vi "TrapControllers.vi"() -> ()   [LabVIEW 2016]
doc: "I. Description:\nThis example demonstrates how to continuously output a waveform using an internal sample clock. The automatic regeneration of data has been disabled, so new data has to be provided throughout the duration of the continuous Analog Output operation. This allows the generation of any arbitrary frequency as this VI computes new data for each iteration of the loop, maintaining phase continuity of the signal. The regeneration of data has also been adjusted so that the newest data is output as quickly as possible; thus reducing the lag between the changing of the data and the output of that data.\n\nII. Instructions for Running:\n1. Select the Physical Channel to correspond to where your signal is output on the DAQ device.\n2. Enter the Minimum and Maximum Voltage range.\n3. Specify the desired Sample Clock Rate of the output Waveform. Higher sample clock rates will produce a smoother waveform.\n4. Manually specify the Analog Output buffer size, in number of samples. A larger buffer would help non-regenerative operations avoid errors due to occasional high CPU load. \nNote: \nThe Analog Output buffer has to be at least as big as the amount of data being written to the board per iteration. The recommended buffer size would be at least twice the amount of data being written to the board per iteration.\n5. Enter the Waveform Information. See the documentation of the Basic Function Generator SubVI for information on each parameter.\n\nIII. Block Diagram Steps:\n1. Create an Analog Output Voltage channel.\n2. Configure the task to prohibit the automatic regeneration of data.\n2a. Set the transfer condition to Less than Full. Allows for more rapid updates of Output Buffer.\n3. Call the DAQmx (Sample Clock) VI to set the sample clock rate. Additionally, set the sample mode to Continuous.\n4. Read the actual sample clock rate (eventually coerced depending on the hardware used). \n5. Compute the desired waveform, using the buffer size and the actual update rate. This VI keeps track of the phase of the waveform to ensure that the generated signal is continuous.\n6. Write the waveform to the output buffer. \n7a. Call the Start VI. This is only needed when the loop is executed for the first time.\n7b. Do nothing.\n8. Loop continuously until user presses the Stop button. Every iteration computes and writes a new waveform to the buffer.\n9. Call the Clear Task VI to clear the Task.\n10. Use the popup dialog box to display an error or warning if any.\n\nIV. I/O Connections Overview:\nMake sure your signal output terminal matches the Physical Channel I/O Control. For further connection information, refer to your hardware reference manual."
uses:
  TrapControllers/PI_PZT controller/PZT_oscillation_stop.vi
panel:
  out "PZT_manual_on":bool
  in  "PZT_oscillation_stop":bool
  out "Loop stop":bool
  out "Numeric":i32
  in  "PZT_Amplitude":dbl=10.0 caption="Amp (nm)" min=0.0 max=100.0 step=1.0 format="%.2f"
  in  "PZT_Frequency":dbl=1.0 caption="Freq (Hz)" min=0.0 max=100.0 step=1.0 format="%.2f"
  in  "PZT_Waveform":T1(ring) caption="Waveform"
  in  "PZT_Axis":enum16{"X-axis", "Y-axis", "Z-axis"}(ring) caption="Axis"
  in  "PZT_oscillation_start":bool caption="Start"
  in  "PZTZ_move":i32=15000 caption="Z"
  in  "PZTY_move":i32=25000 caption="Y"
  in  "PZTX_move":i32=25000 caption="X"
  out "PZTZ_Vin":dbl format="%.4f"
  out "PZTY_Vin":dbl format="%.4f"
  out "PZTX_Vin":dbl format="%.4f"
  out "PZT_Z":i32 caption="Z"
  out "PZT_Y":i32 caption="Y"
  out "PZT_X":i32 caption="X"
  in  "PZT_Move":bool
  out "PZT_Caution":bool caption="Caution"
  in  "PZT_Time":u32=100 caption="Time \n(ms)" max=1000 step=1
  in  "PZT_Step":i32=10 caption="Step \n(nm)" min=0 max=1000 step=1
  in  "PZT_Center":bool
  in  "PZT_Z-":bool
  in  "PZT_Z+":bool
  in  "PZT_Y-":bool
  in  "PZT_Y+":bool
  in  "PZT_X+":bool
  in  "PZT_X-":bool
  out "PZT_ON":bool
  in  "PZT_Start":bool
  out "PZT_Num":i32
  in  "PZT_Stop":bool
  in  "stop 5":bool
  out "Numeric 5":i32
  in  "OK Button 6":bool
  out "OK Button 5":bool
  out "OK Button 4":bool
  in  "stop 2":bool
  out "Numeric 4":i32
  in  "OK Button 2":bool
  in  "STOP":bool
  # "Stop sub-programs first >> STOP PROGRAM"
  # "Servo should be ON."
  # "Manual"
  # "Oscillation"
  # "LED"
  # "Trap Laser"
  # "Move to"
  # "Pos (nm)"
  # "Vin (V)"
  # "PZT"
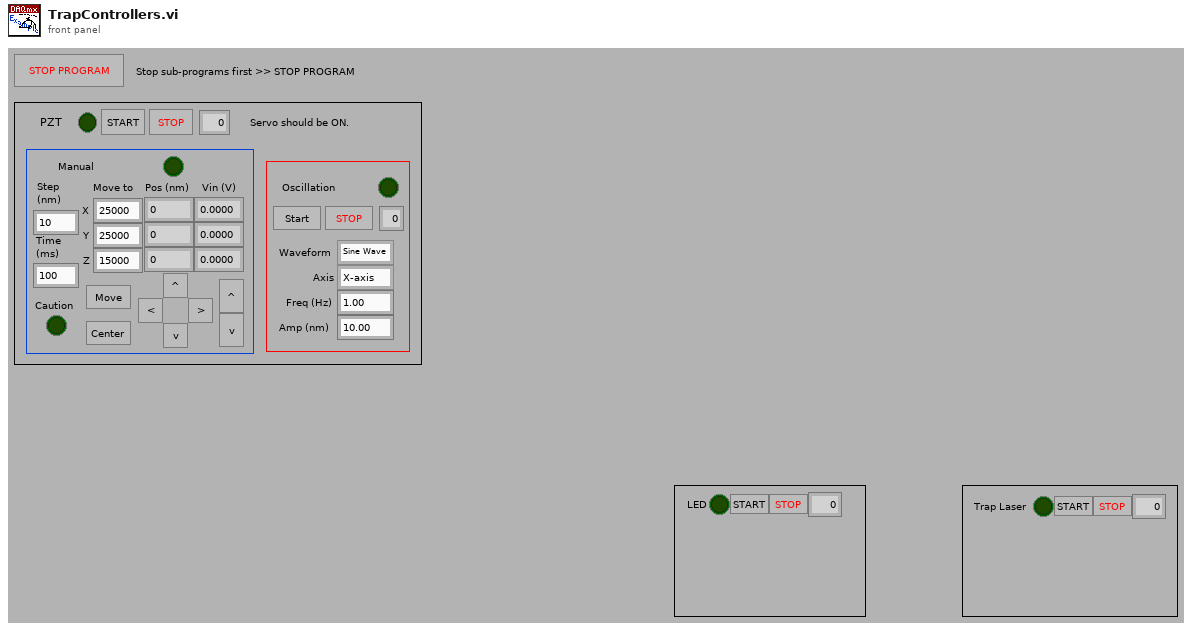
[diagram p1: front panel]
types:
  T1 = enum16{"Sine Wave", "Triangle Wave", "Square Wave", "Sawtooth Wave"}
  T2 = cluster{"PZT_X":i32, "PZT_Y":i32, "PZT_Z":i32, "PZT_Step":i32}
  T3 = typedef "eventvkey.ctl" = enum16{"ASCII", "Enter", "Return", "Shift", "Ctrl", "Alt", "Cmd", "Opt", "Caps", "NumLock", "Clear", "Break", "Up", "Down", "Left", "Right", "Insert", "Delete", "Home", "End", "PageUp", "PageDown", "Escape", "Help", "Pause", "ScrollLock", "F1", "F2", "F3", "F4", "F5", "F6", "F7", "F8", "F9", "F10", "F11", "F12", "F13", "F14", "F15", "F16", "F17", "F18", "F19", "F20", "F21", "F22", "F23", "F24", "Play", "VolumeUp", "VolumeDown", "Mute", "Two Byte Char"}
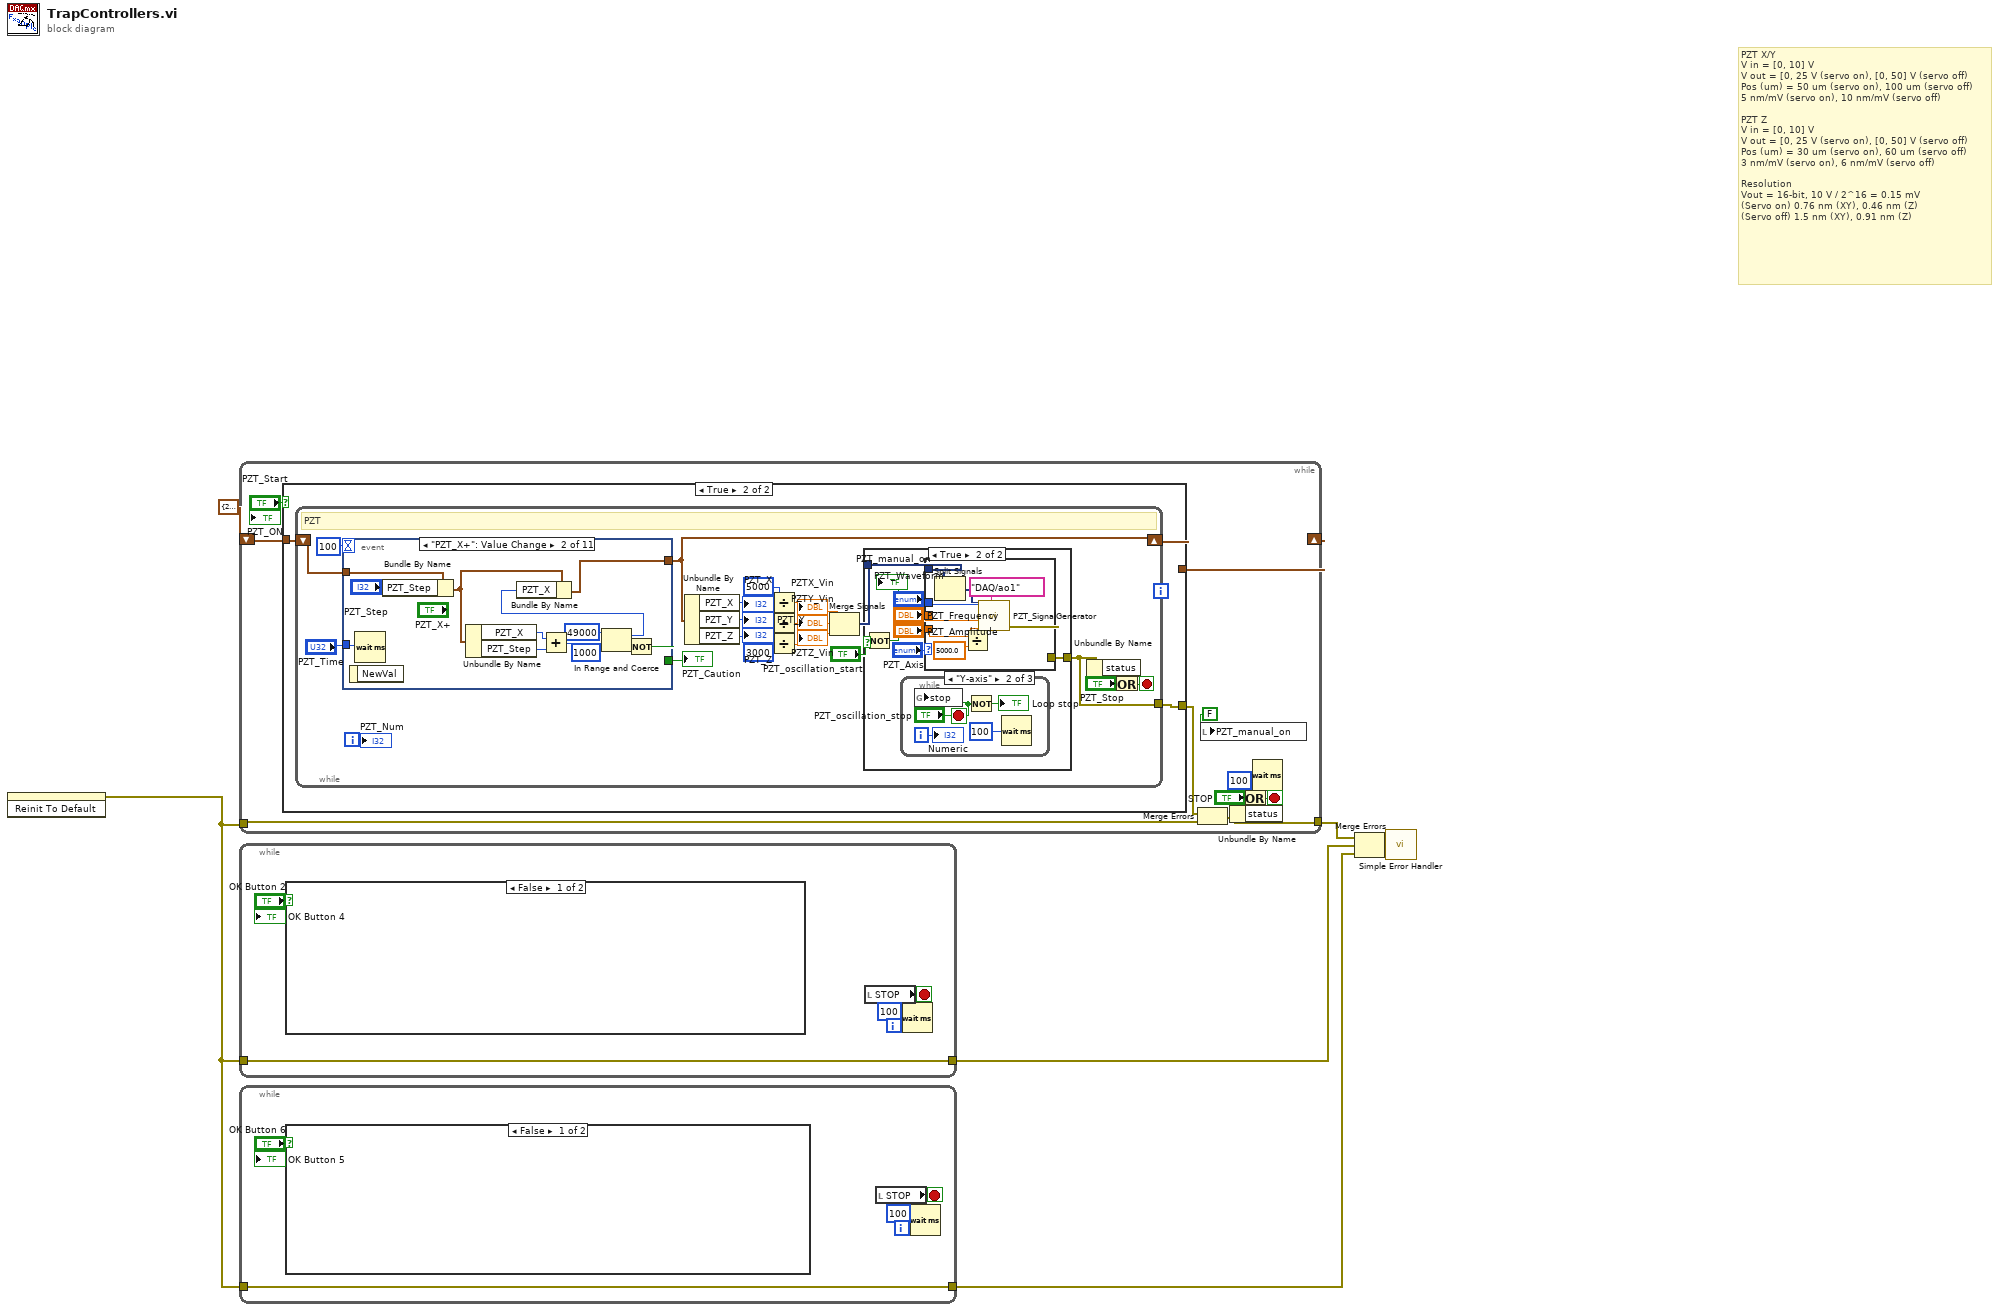
[diagram p0: block diagram]
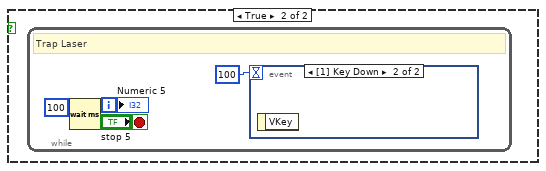
[diagram p2: hidden frame]
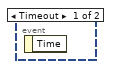
[diagram p3: hidden frame]
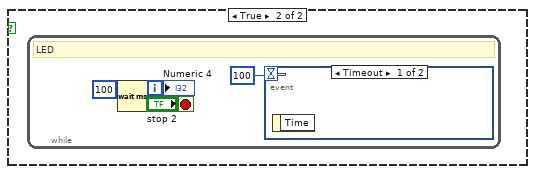
[diagram p4: hidden frame]
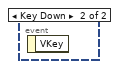
[diagram p5: hidden frame]
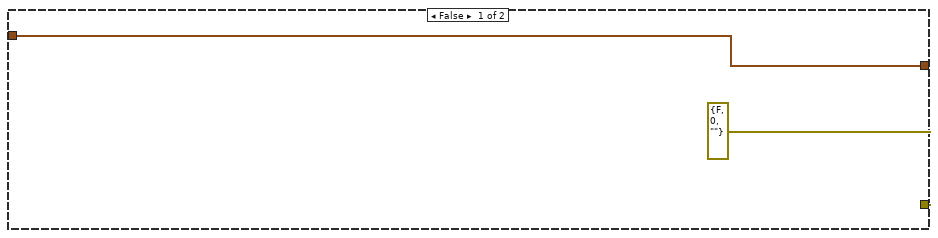
[diagram p6: hidden frame]
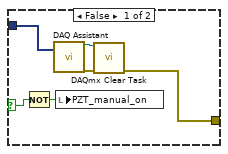
[diagram p7: hidden frame]
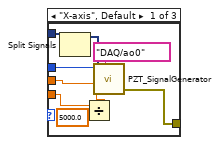
[diagram p8: hidden frame]
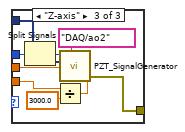
[diagram p9: hidden frame]
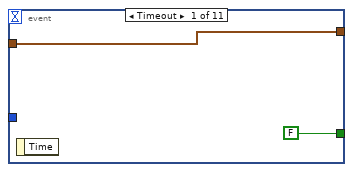
[diagram p10: hidden frame]
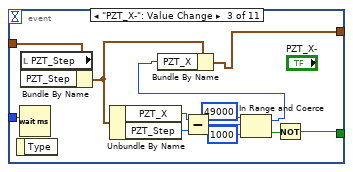
[diagram p11: hidden frame]
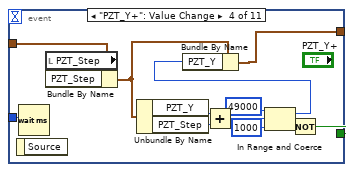
[diagram p12: hidden frame]
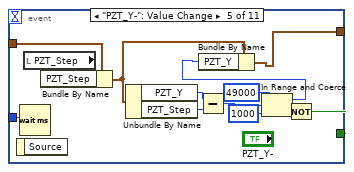
[diagram p13: hidden frame]
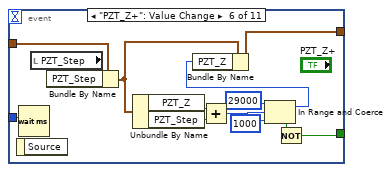
[diagram p14: hidden frame]
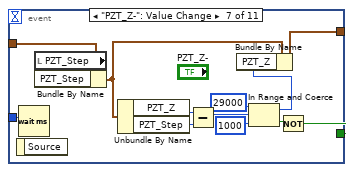
[diagram p15: hidden frame]
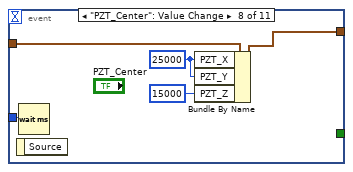
[diagram p16: hidden frame]
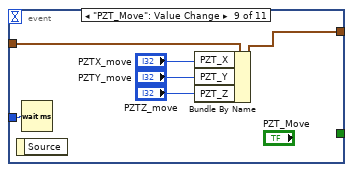
[diagram p17: hidden frame]
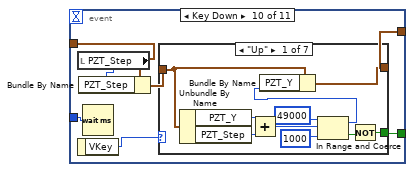
[diagram p18: hidden frame]
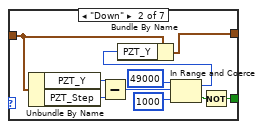
[diagram p19: hidden frame]
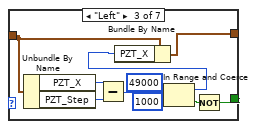
[diagram p20: hidden frame]
diagram:
  # "PZT X/Y\nV in = [0, 10] V\nV out = [0, 25 V (servo on), [0, 50] V (servo off)\nPos (um) = 50 um (servo on), 100 um (servo off)\n5 nm/mV (servo on), 10 nm/mV (servo off)\n\nPZT Z\nV in = [0, 10] V\nV out = [0, 25 V (servo on), [0, 50] V (servo off)\nPos (um) = 30 um (servo on), 60 um (servo off)\n3 nm/mV (servo on), 6 nm/mV (servo off)\n\nResolution\nVout = 16-bit, 10 V / 2^16 = 0.15 mV\n(Servo on) 0.76 nm (XY), 0.46 nm (Z)\n(Servo off) 1.5 nm (XY), 0.91 nm (Z)"
  n1 = invoke on="STOP" class="Bool (strict)" method="Reinit To Default"() -> (error out=w2:errorcluster)  [unwired: 3 in, 2 out]
  n2 = while {
    shift-right: [w16] -> _
    shift-left: T2 {"PZT_X"=25000, "PZT_Y"=25000, "PZT_Z"=15000, "PZT_Step"=10} ("output cluster") -> [w17]
    tunnel: [w11] -> w3
    tunnel: w2 -> [w12]
    stop <- w14 stop-if-true
    n3 = case shown="True" "PZT_Start" {
      tunnel: w17 -> [w19 w22]
      tunnel: [w19 w21] -> w16
      tunnel: [errorcluster {"status"=FALSE, "code"=0, "source"=""} ("error out") w20] -> w13
      frame False {
      }
      frame True {
        n4 = while "Event Handle Loop" {
          shift-right: [w41] -> w21
          shift-left: w22 -> [w28]
          tunnel: [w30] -> w20
          i -> [w42]
          stop <- w32 stop-if-true
          w37 = 5000 ("y")
          # "PZT"
          n5 = event shown="[1] \"PZT_X+\": Value Change" {
            selector: _ -> [_ _ _ _ _ _ _ _ _ _ _]
            dyn-events: _ -> [_ _ _ _ _ _ _ _ _ _ _]
            timeout: 100 -> [_ _ _ _ _ _ _ _ _ _ _]
            tunnel: w28 -> [w89 w98 w112 w125 w138 w151 w164 w172 w178 w184 w253]
            tunnel: [w89 w99 w113 w126 w139 w152 w165 w171 w177 w181 w250] -> w41
            tunnel: [FALSE w91 w106 w118 w133 w143 w156 _ _ w180 w249] -> w39
            tunnel: "PZT_Time" -> [_ w90 w103 w116 w129 w142 w155 w168 w173 w179 w248]
            event Timeout {
              n6 = event-data() -> ()  [unwired: 1 in, 1 out]
            }
            event "PZT_X+": Value Change {
              n7 = event-data() -> ()  [unwired: 1 in, 1 out]
              n8 = Wait (ms)(milliseconds to wait=w90) -> ()  [unwired: 1 out]
              n9 = Bundle By Name(cluster=w98, "PZT_Step"="PZT_Step") -> (w97:T2)
              n10 = Unbundle By Name(w97) -> ("PZT_X"=w101:i32, "PZT_Step"=w100:i32)
              n11 = Add(x=w101, y=w100) -> (x+y=w94:i32)
              n12 = In Range and Coerce(upper limit=49000, x=w94, lower limit=1000) -> (coerced(x)=w93:i32, In Range?=w92:bool)
              n13 = Bundle By Name(cluster=w97, "PZT_X"=w93) -> (w99:T2)
              n14 = Not(x=w92) -> (.not. x?=w91:bool)
            }
            event "PZT_X-": Value Change {
              n15 = event-data() -> ()  [unwired: 1 in, 1 out]
              n16 = Wait (ms)(milliseconds to wait=w103) -> ()  [unwired: 1 out]
              n17 = local read "PZT_Step"() -> (w110:i32)
              n18 = Bundle By Name(cluster=w112, "PZT_Step"=w110) -> (w111:T2)
              n19 = Unbundle By Name(w111) -> ("PZT_X"=w115:i32, "PZT_Step"=w114:i32)
              n20 = Subtract(x=w115, y=w114) -> (x-y=w107:i32)
              n21 = In Range and Coerce(upper limit=49000, x=w107, lower limit=1000) -> (coerced(x)=w105:i32, In Range?=w108:bool)
              n22 = Bundle By Name(cluster=w111, "PZT_X"=w105) -> (w113:T2)
              n23 = Not(x=w108) -> (.not. x?=w106:bool)
            }
            event "PZT_Y+": Value Change {
              n24 = event-data() -> ()  [unwired: 1 in, 1 out]
              n25 = Wait (ms)(milliseconds to wait=w116) -> ()  [unwired: 1 out]
              n26 = local read "PZT_Step"() -> (w123:i32)
              n27 = Bundle By Name(cluster=w125, "PZT_Step"=w123) -> (w124:T2)
              n28 = Unbundle By Name(w124) -> ("PZT_Y"=w128:i32, "PZT_Step"=w127:i32)
              n29 = Add(x=w128, y=w127) -> (x+y=w120:i32)
              n30 = In Range and Coerce(upper limit=49000, x=w120, lower limit=1000) -> (coerced(x)=w119:i32, In Range?=w121:bool)
              n31 = Bundle By Name(cluster=w124, "PZT_Y"=w119) -> (w126:T2)
              n32 = Not(x=w121) -> (.not. x?=w118:bool)
            }
            event "PZT_Y-": Value Change {
              n33 = event-data() -> ()  [unwired: 1 in, 1 out]
              n34 = Wait (ms)(milliseconds to wait=w129) -> ()  [unwired: 1 out]
              n35 = local read "PZT_Step"() -> (w136:i32)
              n36 = Bundle By Name(cluster=w138, "PZT_Step"=w136) -> (w137:T2)
              n37 = Unbundle By Name(w137) -> ("PZT_Y"=w141:i32, "PZT_Step"=w140:i32)
              n38 = Subtract(x=w141, y=w140) -> (x-y=w131:i32)
              n39 = In Range and Coerce(upper limit=49000, x=w131, lower limit=1000) -> (coerced(x)=w130:i32, In Range?=w134:bool)
              n40 = Bundle By Name(cluster=w137, "PZT_Y"=w130) -> (w139:T2)
              n41 = Not(x=w134) -> (.not. x?=w133:bool)
            }
            event "PZT_Z+": Value Change {
              n42 = event-data() -> ()  [unwired: 1 in, 1 out]
              n43 = Wait (ms)(milliseconds to wait=w142) -> ()  [unwired: 1 out]
              n44 = local read "PZT_Step"() -> (w149:i32)
              n45 = Bundle By Name(cluster=w151, "PZT_Step"=w149) -> (w150:T2)
              n46 = Unbundle By Name(w150) -> ("PZT_Z"=w154:i32, "PZT_Step"=w153:i32)
              n47 = Add(x=w154, y=w153) -> (x+y=w146:i32)
              n48 = In Range and Coerce(upper limit=29000, x=w146, lower limit=1000) -> (coerced(x)=w144:i32, In Range?=w147:bool)
              n49 = Bundle By Name(cluster=w150, "PZT_Z"=w144) -> (w152:T2)
              n50 = Not(x=w147) -> (.not. x?=w143:bool)
            }
            event "PZT_Z-": Value Change {
              n51 = event-data() -> ()  [unwired: 1 in, 1 out]
              n52 = Wait (ms)(milliseconds to wait=w155) -> ()  [unwired: 1 out]
              n53 = local read "PZT_Step"() -> (w162:i32)
              n54 = Bundle By Name(cluster=w164, "PZT_Step"=w162) -> (w163:T2)
              n55 = Unbundle By Name(w163) -> ("PZT_Z"=w167:i32, "PZT_Step"=w166:i32)
              n56 = Subtract(x=w167, y=w166) -> (x-y=w159:i32)
              n57 = In Range and Coerce(upper limit=29000, x=w159, lower limit=1000) -> (coerced(x)=w157:i32, In Range?=w160:bool)
              n58 = Bundle By Name(cluster=w163, "PZT_Z"=w157) -> (w165:T2)
              n59 = Not(x=w160) -> (.not. x?=w156:bool)
            }
            event "PZT_Center": Value Change {
              w170 = 25000 ("PZT_X")
              n60 = event-data() -> ()  [unwired: 1 in, 1 out]
              n61 = Wait (ms)(milliseconds to wait=w168) -> ()  [unwired: 1 out]
              n62 = Bundle By Name(cluster=w172, "PZT_X"=w170, "PZT_Y"=w170, "PZT_Z"=15000) -> (w171:T2)
            }
            event "PZT_Move": Value Change {
              n63 = event-data() -> ()  [unwired: 1 in, 1 out]
              n64 = Wait (ms)(milliseconds to wait=w173) -> ()  [unwired: 1 out]
              n65 = Bundle By Name(cluster=w178, "PZT_X"="PZTX_move", "PZT_Y"="PZTY_move", "PZT_Z"="PZTZ_move") -> (w177:T2)
            }
            event Key Down {
              n66 = local read "PZT_Step"() -> (w183:i32)
              n67 = event-data() -> ("VKey"=w185:T3)  [unwired: 1 in]
              n68 = Bundle By Name(cluster=w184, "PZT_Step"=w183) -> (w182:T2)
              n69 = Wait (ms)(milliseconds to wait=w179) -> ()  [unwired: 1 out]
              n70 = case shown="\"Up\"" w185 {
                tunnel: w182 -> [w193 w203 w213 w223 w233 w243 w247]
                tunnel: [w192 w202 w212 w222 w232 w242 w247] -> w181
                tunnel: [w187 w198 w208 w218 w228 w238 FALSE] -> w180
                frame "Up" {
                  n71 = Unbundle By Name(w193) -> ("PZT_Y"=w195:i32, "PZT_Step"=w194:i32)
                  n72 = Add(x=w195, y=w194) -> (x+y=w189:i32)
                  n73 = In Range and Coerce(upper limit=49000, x=w189, lower limit=1000) -> (coerced(x)=w186:i32, In Range?=w190:bool)
                  n74 = Bundle By Name(cluster=w193, "PZT_Y"=w186) -> (w192:T2)
                  n75 = Not(x=w190) -> (.not. x?=w187:bool)
                }
                frame "Down" {
                  n76 = Unbundle By Name(w203) -> ("PZT_Y"=w205:i32, "PZT_Step"=w204:i32)
                  n77 = Subtract(x=w205, y=w204) -> (x-y=w197:i32)
                  n78 = In Range and Coerce(upper limit=49000, x=w197, lower limit=1000) -> (coerced(x)=w196:i32, In Range?=w200:bool)
                  n79 = Bundle By Name(cluster=w203, "PZT_Y"=w196) -> (w202:T2)
                  n80 = Not(x=w200) -> (.not. x?=w198:bool)
                }
                frame "Left" {
                  n81 = Unbundle By Name(w213) -> ("PZT_X"=w215:i32, "PZT_Step"=w214:i32)
                  n82 = Subtract(x=w215, y=w214) -> (x-y=w207:i32)
                  n83 = In Range and Coerce(upper limit=49000, x=w207, lower limit=1000) -> (coerced(x)=w206:i32, In Range?=w210:bool)
                  n84 = Bundle By Name(cluster=w213, "PZT_X"=w206) -> (w212:T2)
                  n85 = Not(x=w210) -> (.not. x?=w208:bool)
                }
                frame "Right" {
                  n86 = Unbundle By Name(w223) -> ("PZT_X"=w225:i32, "PZT_Step"=w224:i32)
                  n87 = Add(x=w225, y=w224) -> (x+y=w217:i32)
                  n88 = In Range and Coerce(upper limit=49000, x=w217, lower limit=1000) -> (coerced(x)=w216:i32, In Range?=w220:bool)
                  n89 = Bundle By Name(cluster=w223, "PZT_X"=w216) -> (w222:T2)
                  n90 = Not(x=w220) -> (.not. x?=w218:bool)
                }
                frame "PageUp" {
                  n91 = Unbundle By Name(w233) -> ("PZT_Z"=w235:i32, "PZT_Step"=w234:i32)
                  n92 = Add(x=w235, y=w234) -> (x+y=w227:i32)
                  n93 = In Range and Coerce(upper limit=29000, x=w227, lower limit=1000) -> (coerced(x)=w226:i32, In Range?=w230:bool)
                  n94 = Bundle By Name(cluster=w233, "PZT_Z"=w226) -> (w232:T2)
                  n95 = Not(x=w230) -> (.not. x?=w228:bool)
                }
                frame "PageDown" {
                  n96 = Unbundle By Name(w243) -> ("PZT_Z"=w245:i32, "PZT_Step"=w244:i32)
                  n97 = Subtract(x=w245, y=w244) -> (x-y=w237:i32)
                  n98 = In Range and Coerce(upper limit=29000, x=w237, lower limit=1000) -> (coerced(x)=w236:i32, In Range?=w240:bool)
                  n99 = Bundle By Name(cluster=w243, "PZT_Z"=w236) -> (w242:T2)
                  n100 = Not(x=w240) -> (.not. x?=w238:bool)
                }
                frame Default {
                }
              }
            }
            event Key Repeat {
              n101 = local read "PZT_Step"() -> (w252:i32)
              n102 = event-data() -> ("VKey"=w254:T3)  [unwired: 1 in]
              n103 = Bundle By Name(cluster=w253, "PZT_Step"=w252) -> (w251:T2)
              n104 = Wait (ms)(milliseconds to wait=w248) -> ()  [unwired: 1 out]
              n105 = case shown="\"Right\"" w254 {
                tunnel: w251 -> [w262 w272 w282 w292 w302 w312 w316]
                tunnel: [w261 w271 w281 w291 w301 w311 w316] -> w250
                tunnel: [w255 w265 w275 w285 w295 w305 FALSE] -> w249
                frame "Up" {
                  n106 = Unbundle By Name(w262) -> ("PZT_Y"=w264:i32, "PZT_Step"=w263:i32)
                  n107 = Add(x=w264, y=w263) -> (x+y=w260:i32)
                  n108 = In Range and Coerce(upper limit=49000, x=w260, lower limit=1000) -> (coerced(x)=w259:i32, In Range?=w256:bool)
                  n109 = Bundle By Name(cluster=w262, "PZT_Y"=w259) -> (w261:T2)
                  n110 = Not(x=w256) -> (.not. x?=w255:bool)
                }
                frame "Down" {
                  n111 = Unbundle By Name(w272) -> ("PZT_Y"=w274:i32, "PZT_Step"=w273:i32)
                  n112 = Subtract(x=w274, y=w273) -> (x-y=w270:i32)
                  n113 = In Range and Coerce(upper limit=49000, x=w270, lower limit=1000) -> (coerced(x)=w267:i32, In Range?=w266:bool)
                  n114 = Bundle By Name(cluster=w272, "PZT_Y"=w267) -> (w271:T2)
                  n115 = Not(x=w266) -> (.not. x?=w265:bool)
                }
                frame "Left" {
                  n116 = Unbundle By Name(w282) -> ("PZT_X"=w284:i32, "PZT_Step"=w283:i32)
                  n117 = Subtract(x=w284, y=w283) -> (x-y=w280:i32)
                  n118 = In Range and Coerce(upper limit=49000, x=w280, lower limit=1000) -> (coerced(x)=w277:i32, In Range?=w276:bool)
                  n119 = Bundle By Name(cluster=w282, "PZT_X"=w277) -> (w281:T2)
                  n120 = Not(x=w276) -> (.not. x?=w275:bool)
                }
                frame "Right" {
                  n121 = Unbundle By Name(w292) -> ("PZT_X"=w294:i32, "PZT_Step"=w293:i32)
                  n122 = Add(x=w294, y=w293) -> (x+y=w290:i32)
                  n123 = In Range and Coerce(upper limit=49000, x=w290, lower limit=1000) -> (coerced(x)=w287:i32, In Range?=w286:bool)
                  n124 = Bundle By Name(cluster=w292, "PZT_X"=w287) -> (w291:T2)
                  n125 = Not(x=w286) -> (.not. x?=w285:bool)
                }
                frame "PageUp" {
                  n126 = Unbundle By Name(w302) -> ("PZT_Z"=w304:i32, "PZT_Step"=w303:i32)
                  n127 = Add(x=w304, y=w303) -> (x+y=w300:i32)
                  n128 = In Range and Coerce(upper limit=29000, x=w300, lower limit=1000) -> (coerced(x)=w297:i32, In Range?=w296:bool)
                  n129 = Bundle By Name(cluster=w302, "PZT_Z"=w297) -> (w301:T2)
                  n130 = Not(x=w296) -> (.not. x?=w295:bool)
                }
                frame "PageDown" {
                  n131 = Unbundle By Name(w312) -> ("PZT_Z"=w314:i32, "PZT_Step"=w313:i32)
                  n132 = Subtract(x=w314, y=w313) -> (x-y=w310:i32)
                  n133 = In Range and Coerce(upper limit=29000, x=w310, lower limit=1000) -> (coerced(x)=w307:i32, In Range?=w306:bool)
                  n134 = Bundle By Name(cluster=w312, "PZT_Z"=w307) -> (w311:T2)
                  n135 = Not(x=w306) -> (.not. x?=w305:bool)
                }
                frame Default {
                }
              }
            }
          }
          "PZT_Caution" <- w39
          n136 = Unbundle By Name(w41) -> ("PZT_X"=w38:i32, "PZT_Y"=w36:i32, "PZT_Z"=w35:i32)
          "PZT_X" <- w38
          "PZT_Y" <- w36
          "PZT_Z" <- w35
          n137 = Divide(x=w38, y=w37) -> (x/y=w27:dbl)
          "PZTX_Vin" <- w27
          n138 = Divide(x=w36, y=w37) -> (x/y=w26:dbl)
          "PZTY_Vin" <- w26
          n139 = Divide(x=w35, y=3000) -> (x/y=w25:dbl)
          "PZTZ_Vin" <- w25
          n140 = Merge Signals(w27, w26, w25) -> (w24:dynamicdata)
          n141 = case shown="True" "PZT_oscillation_start" {
            selector: "PZT_oscillation_start" -> [w43 w49]
            tunnel: [w45 w54] -> w30
            tunnel: w24 -> [w48 w55]
            frame False {
              n142 = Not(x=w43) -> (.not. x?=w44:bool)
              n143 = call "DAQ Assistant"("data"=w48) -> ("task out"=w46:refnum<k21>, "error out"=w47:errorcluster)  [unwired: 17 in]
              n144 = local write "PZT_manual_on"(w44) -> ()
              n145 = call <vilib>:"DAQmx Clear Task.vi"("task in"=w46, "error in"=w47) -> ("error out"=w45:errorcluster)  [unwired: 13 in]
            }
            frame True {
              n146 = Not(x=w49) -> (.not. x?=→"PZT_manual_on":bool)
              n147 = while {
                i -> [w60]
                stop <- "PZT_oscillation_stop" stop-if-true
                n148 = global write "PZT_oscillation_stop.vi" "stop"("PZT_oscillation_stop") -> ()
                n149 = Not(x="PZT_oscillation_stop") -> (.not. x?=→"Loop stop":bool)
                n150 = Wait (ms)(milliseconds to wait=u32 100) -> ()  [unwired: 1 out]
                "Numeric" <- w60
              }
              n151 = case shown="\"Y-axis\"" "PZT_Axis" {
                tunnel: w55 -> [w67 w76 w85]
                tunnel: [w68 w77 w86] -> w54
                tunnel: "PZT_Waveform" -> [w65 w74 w83]
                tunnel: "PZT_Frequency" -> [w64 w75 w84]
                tunnel: "PZT_Amplitude" -> [w63 w71 w80]
                frame "X-axis", Default {
                  n152 = Split Signals(w67) -> (w66:dynamicdata)  [unwired: 3 in, 2 out]
                  n153 = Divide(x=w63, y=5000.0) -> (x/y=w62:dbl)
                  n154 = call "PZT_SignalGenerator.vi"("Waveform Type"=w65, "Physical Channels"=tag "DAQ/ao0", "Offset"=w66, "Frequency"=w64, "Amplitude"=w62) -> ("error out"=w68:errorcluster)  [unwired: 2 in, 1 out]
                }
                frame "Y-axis" {
                  n155 = Split Signals(w76) -> (w70:dynamicdata)  [unwired: 3 in, 2 out]
                  n156 = Divide(x=w71, y=5000.0) -> (x/y=w72:dbl)
                  n157 = call "PZT_SignalGenerator.vi"("Waveform Type"=w74, "Physical Channels"=tag "DAQ/ao1", "Offset"=w70, "Frequency"=w75, "Amplitude"=w72) -> ("error out"=w77:errorcluster)  [unwired: 2 in, 1 out]
                }
                frame "Z-axis" {
                  n158 = Split Signals(w85) -> (w82:dynamicdata)  [unwired: 3 in, 2 out]
                  n159 = Divide(x=w80, y=3000.0) -> (x/y=w79:dbl)
                  n160 = call "PZT_SignalGenerator.vi"("Waveform Type"=w83, "Physical Channels"=tag "DAQ/ao2", "Offset"=w82, "Frequency"=w84, "Amplitude"=w79) -> ("error out"=w86:errorcluster)  [unwired: 2 in, 1 out]
                }
              }
            }
          }
          n161 = Unbundle By Name(w30) -> ("status"=w31:bool)
          n162 = Or(x=w31, y="PZT_Stop") -> (x .or. y?=w32:bool)
          "PZT_Num" <- w42
        }
      }
    }
    n163 = Merge Errors(w13, w12) -> (w11:errorcluster)
    n164 = local write "PZT_manual_on"(FALSE) -> ()
    n165 = Unbundle By Name(w11) -> ("status"=w9:bool)
    n166 = Or(x="STOP", y=w9) -> (x .or. y?=w14:bool)
    n167 = Wait (ms)(milliseconds to wait=u32 100) -> ()  [unwired: 1 out]
    "PZT_ON" <- "PZT_Start"
  }
  n168 = while {
    tunnel: w2 -> [w318]
    tunnel: [w318] -> w5
    stop <- w319 stop-if-true
    n169 = case shown="False" "OK Button 2" {
      frame False {
      }
      frame True {
        n170 = while "Event Handle Loop" {
          i -> [w323]
          stop <- "stop 2" stop-if-true
          # "LED"
          n171 = Wait (ms)(milliseconds to wait=u32 100) -> ()  [unwired: 1 out]
          n172 = event shown="[0] Timeout" {
            selector: _ -> [_ _]
            dyn-events: _ -> [_ _]
            timeout: 100 -> [_ _]
            event Timeout {
              n173 = event-data() -> ()  [unwired: 1 in, 1 out]
            }
            event Key Down {
              n174 = event-data() -> ()  [unwired: 1 in, 1 out]
            }
          }
          "Numeric 4" <- w323
        }
      }
    }
    n175 = local read "STOP"() -> (w319:bool)
    n176 = Wait (ms)(milliseconds to wait=u32 100) -> ()  [unwired: 1 out]
    "OK Button 4" <- "OK Button 2"
  }
  n177 = while {
    tunnel: w2 -> [w326]
    tunnel: [w326] -> w4
    stop <- w327 stop-if-true
    n178 = case shown="False" "OK Button 6" {
      frame False {
      }
      frame True {
        n179 = while "Event Handle Loop" {
          i -> [w330]
          stop <- "stop 5" stop-if-true
          # "Trap Laser"
          n180 = Wait (ms)(milliseconds to wait=u32 100) -> ()  [unwired: 1 out]
          n181 = event shown="[1] Key Down" {
            selector: _ -> [_ _]
            dyn-events: _ -> [_ _]
            timeout: 100 -> [_ _]
            event Timeout {
              n182 = event-data() -> ()  [unwired: 1 in, 1 out]
            }
            event Key Down {
              n183 = event-data() -> ()  [unwired: 1 in, 1 out]
            }
          }
          "Numeric 5" <- w330
        }
      }
    }
    n184 = local read "STOP"() -> (w327:bool)
    n185 = Wait (ms)(milliseconds to wait=u32 100) -> ()  [unwired: 1 out]
    "OK Button 5" <- "OK Button 6"
  }
  n186 = Merge Errors(w3, w5, w4) -> (w6:errorcluster)
  n187 = call <vilib>:"Simple Error Handler.vi"("error in (no error)"=w6) -> ()  [unwired: 4 in, 5 out]
